vi "短日期时间转长日期格式.vi"(10 "table输入":string(combo), 11 "data":string[][](table)) -> (3 "输出数组":string[][](array[string]))   [LabVIEW 2016, in "数据传输系统.lvlib"]
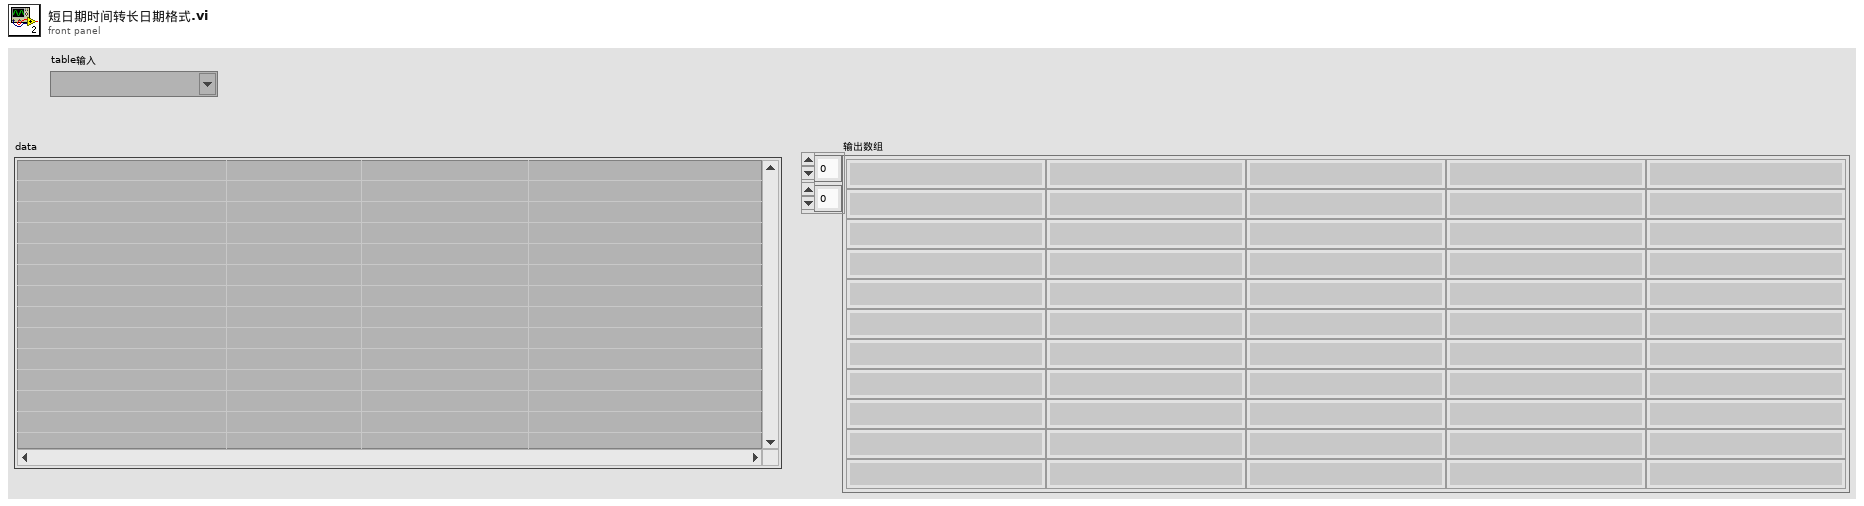
[diagram p1: front panel]
types:
  T1 = typedef "LVDateTimeRec.ctl" = cluster{"秒数的小数部分":dbl, "秒":i32, "分":i32, "时":i32, "日":i32, "月":i32, "年":i32, "天数（周）":i32, "天数（年）":i32, "DST":i32}
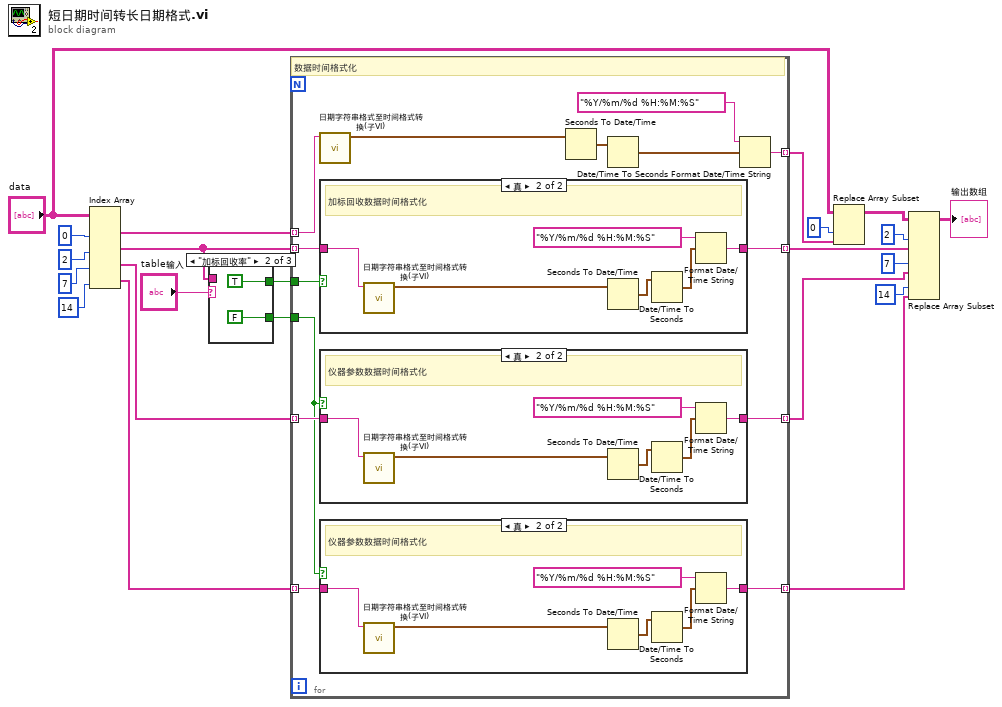
[diagram p0: block diagram]
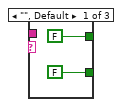
[diagram p5: hidden frame]
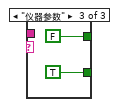
[diagram p6: hidden frame]
diagram:
  n1 = Index Array(array="data", index (col) #1=0 ("禁用的索引 (列)"), index (col) #2=2 ("索引 (列)"), index (col) #3=7 ("索引 (列)"), index (col) #4=14 ("索引 (列)")) -> (element #1=w11:string[], element #2=w10:string[], element #3=w7:string[], element #4=w6:string[])  [unwired: 4 in]
  n2 = case shown="\"加标回收率\"" "table输入" {
    tunnel: [FALSE TRUE FALSE] -> w12
    tunnel: w10 -> [_ _ _]
    tunnel: [FALSE FALSE TRUE] -> w5
    frame "", Default {
    }
    frame "加标回收率" {
    }
    frame "仪器参数" {
    }
  }
  n3 = for {
    tunnel: [w38] -> w18 mode=indexing
    tunnel: [w37] -> w14 mode=indexing
    tunnel: w12 -> [w36]
    tunnel: w11 -> [w35] mode=indexing
    tunnel: w10 -> [w34] mode=indexing
    tunnel: w7 -> [w33] mode=indexing
    tunnel: w6 -> [w32] mode=indexing
    tunnel: w5 -> [w31]
    tunnel: [w30] -> w2 mode=indexing
    tunnel: [w29] -> w1 mode=indexing
    # "数据时间格式化"
    n4 = call "日期字符串格式至时间格式转换(子VI).vi"("data[0]"=w35) -> ("time stamp"=w41:timestamp)  [unwired: 10 in]
    n5 = case shown="真" w36 {
      tunnel: [w57 w59] -> w37
      tunnel: w34 -> [w57 w58]
      frame False {
      }
      frame True {
        # "加标回收数据时间格式化"
        n6 = call "日期字符串格式至时间格式转换(子VI).vi"("data[0]"=w58) -> ("time stamp"=w61:timestamp)  [unwired: 10 in]
        n7 = Seconds To Date/Time(time stamp (now)=w61) -> (date time rec=w60:T1)  [unwired: 1 in]
        n8 = Date/Time To Seconds(2:w60) -> (0:w62:timestamp)  [unwired: 1 in]
        n9 = Format Date/Time String(time format string (%c)="%Y/%m/%d %H:%M:%S" ("时间格式字符串(%c)"), seconds (now)=w62) -> (date/time string=w59:string)  [unwired: 1 in]
      }
    }
    n10 = case shown="真" w31 {
      tunnel: [w50 w52] -> w30
      tunnel: w33 -> [w50 w51]
      frame False {
      }
      frame True {
        # "仪器参数数据时间格式化"
        n11 = call "日期字符串格式至时间格式转换(子VI).vi"("data[0]"=w51) -> ("time stamp"=w54:timestamp)  [unwired: 10 in]
        n12 = Seconds To Date/Time(time stamp (now)=w54) -> (date time rec=w53:T1)  [unwired: 1 in]
        n13 = Date/Time To Seconds(2:w53) -> (0:w55:timestamp)  [unwired: 1 in]
        n14 = Format Date/Time String(time format string (%c)="%Y/%m/%d %H:%M:%S" ("时间格式字符串(%c)"), seconds (now)=w55) -> (date/time string=w52:string)  [unwired: 1 in]
      }
    }
    n15 = case shown="真" w31 {
      tunnel: [w43 w45] -> w29
      tunnel: w32 -> [w43 w44]
      frame False {
      }
      frame True {
        # "仪器参数数据时间格式化"
        n16 = call "日期字符串格式至时间格式转换(子VI).vi"("data[0]"=w44) -> ("time stamp"=w47:timestamp)  [unwired: 10 in]
        n17 = Seconds To Date/Time(time stamp (now)=w47) -> (date time rec=w46:T1)  [unwired: 1 in]
        n18 = Date/Time To Seconds(2:w46) -> (0:w48:timestamp)  [unwired: 1 in]
        n19 = Format Date/Time String(time format string (%c)="%Y/%m/%d %H:%M:%S" ("时间格式字符串(%c)"), seconds (now)=w48) -> (date/time string=w45:string)  [unwired: 1 in]
      }
    }
    n20 = Seconds To Date/Time(time stamp (now)=w41) -> (date time rec=w42:T1)  [unwired: 1 in]
    n21 = Date/Time To Seconds(2:w42) -> (0:w40:timestamp)  [unwired: 1 in]
    n22 = Format Date/Time String(time format string (%c)="%Y/%m/%d %H:%M:%S" ("时间格式字符串(%c)"), seconds (now)=w40) -> (date/time string=w38:string)  [unwired: 1 in]
  }
  n23 = Replace Array Subset(array="data", new element=w18, index (col)=0 ("禁用的索引 (列)")) -> (w15:string[][])  [unwired: 1 in]
  n24 = Replace Array Subset(array=w15, new element #1=w14, index (col) #1=2 ("索引 (列)"), new element #2=w2, index (col) #2=7 ("索引 (列)"), new element #3=w1, index (col) #3=14 ("索引 (列)")) -> (→"输出数组":string[][])  [unwired: 3 in]
